vi "(re)create reuse events.vi"(4 "error in (no error)":errorcluster, 5 "Save Menu":refnum<vi>, 6 "Save Button":refnum<vi>, 7 "reuse in":refnum<event-registration>) -> (0 "error out":errorcluster, 3 "reuse":refnum<event-registration>)   [LabVIEW 2014, in "Startup Processes.lvlib"]
uses:
  Startup Processes.lvlib
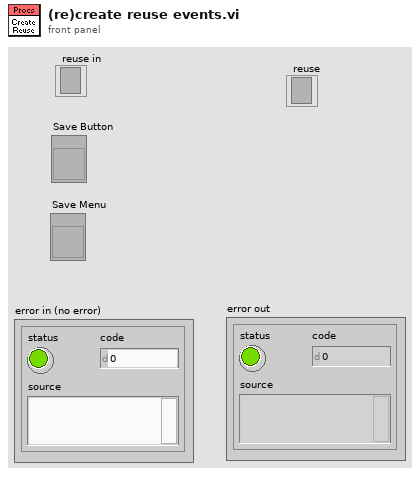
[diagram p1: front panel]
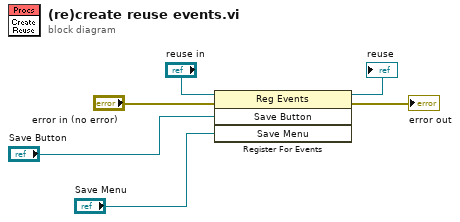
[diagram p0: block diagram]
diagram:
  n1 = register-events(reference="reuse in", error in="error in (no error)", "Save Button", "Save Menu") -> (reference out=→"reuse":refnum<event-registration>, error out=→"error out":errorcluster)
